vi "DEC2BIN.vi"(10 "DECIMAL":dbl[](array[numeric])=[-3.0]) -> (2 "BINARY":string[](array[string]))   [LabVIEW 2021]
panel:
  out "Dec2Bin":string
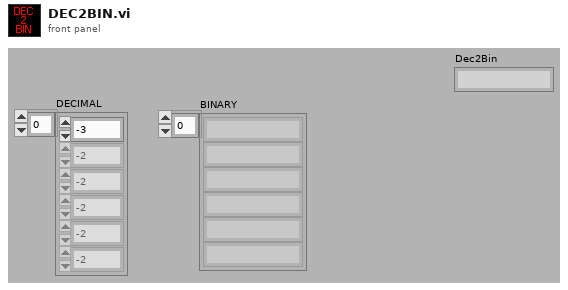
[diagram p1: front panel]
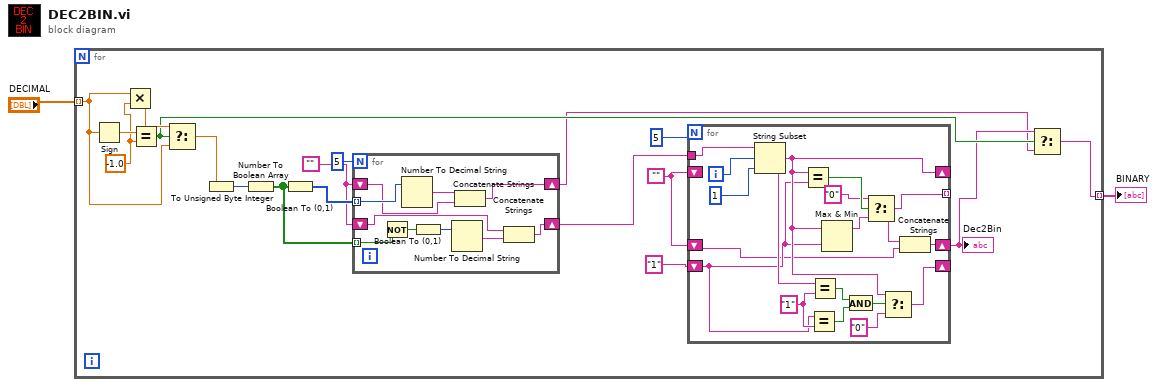
[diagram p0: block diagram]
diagram:
  n1 = for {
    tunnel: "DECIMAL" -> [w16] mode=indexing
    tunnel: [w4] -> w1 mode=indexing
    w8 = ""
    w12 = ""
    w18 = -1.0 ("y")
    n2 = Sign(1:w16) -> (0:w20:dbl)
    n3 = Multiply(x=w16, y=w18) -> (x*y=w17:dbl)
    n4 = Equal?(x=w20, y=w18) -> (x = y?=w7:bool)
    n5 = Select(t=w17, s=w7, f=w16) -> (s? t:f=w15:dbl)
    n6 = To Unsigned Byte Integer(number=w15) -> (unsigned 8bit integer=w19:u8)
    n7 = Number To Boolean Array(number=w19) -> (Boolean array=w13:bool[])
    n8 = Boolean To (0,1)(Boolean=w13) -> (0, 1=w14:i16[])
    n9 = for {
      N: 5 -> [_]
      tunnel: w14 -> [w47] mode=indexing
      shift-right: [w46] -> w5
      shift-left: w12 -> [w38]
      tunnel: w13 -> [w45] mode=indexing
      shift-right: [w40] -> w11
      shift-left: w12 -> [w42]
      n10 = Not(x=w45) -> (.not. x?=w44:bool)
      n11 = Number To Decimal String(number=w47) -> (decimal integer string=w39:string)  [unwired: 1 in]
      n12 = Boolean To (0,1)(Boolean=w44) -> (0, 1=w43:i16)
      n13 = Number To Decimal String(number=w43) -> (decimal integer string=w41:string)  [unwired: 1 in]
      n14 = Concatenate Strings(w39, w38) -> (w46:string)
      n15 = Concatenate Strings(w42, w41) -> (w40:string)
    }
    n16 = for {
      N: 5 -> [_]
      tunnel: w11 -> [w37]
      shift-right: [w27] -> _
      shift-left: w8 -> [_]
      shift-right: [w28] -> _
      shift-left: "1" -> [w26]
      tunnel: [w23] -> _ mode=indexing
      shift-right: [w22] -> w6
      shift-left: w8 -> [w21]
      i -> [w36]
      w33 = "1"
      n17 = String Subset(string=w37, offset (0)=w36, length (rest)=1 ("length (rest)")) -> (substring=w27:string)
      n18 = Equal?(x=w27, y=w26) -> (x = y?=w34:bool)
      n19 = Equal?(x=w26, y=w33) -> (x = y?=w31:bool)
      n20 = Equal?(x=w27, y=w33) -> (x = y?=w32:bool)
      n21 = Max & Min(x=w27, y=w26) -> (max(x,y)=w25:string)  [unwired: 1 out]
      n22 = And(x=w32, y=w31) -> (x .and. y?=w30:bool)
      n23 = Select(t="0", s=w34, f=w25) -> (s? t:f=w23:string)
      n24 = Select(t=w27, s=w30, f="0") -> (s? t:f=w28:string)
      n25 = Concatenate Strings(w23, w21) -> (w22:string)
    }
    "Dec2Bin" <- w6
    n26 = Select(t=w6, s=w7, f=w5) -> (s? t:f=w4:string)
  }
  "BINARY" <- w1
